vi "Repeater.vi"(7 "Name":string="Repeater", 10 "Finish On":T1, 11 "Node In":refnum<class "abs_Node.lvclass">) -> (3 "Node Out":refnum<class "abs_Node.lvclass">)   [LabVIEW 2021, in "BT.lvlib"]
uses:
  BT.lvlib
  abs_Node/abs_Node.lvclass
  Repeater/Support/Finish On - Type.ctl
  Repeater/Repeater.lvclass
  C:/Users/Tim/Documents/LabVIEW/2021/Behaviour Tree/abs_Node/abs_Node.lvclass
  C:/Users/Tim/Documents/LabVIEW/2021/Behaviour Tree/abs_Decorator/abs_Decorator.lvclass
  abs_Node/abs_Node.lvclass/abs_Node.ctl
  abs_Decorator/abs_Decorator.lvclass/abs_Decorator.ctl
  Repeater/Repeater.lvclass/Repeater.ctl
  abs_Node/Properties/Write Name.vi
  abs_Decorator/Properties/Write Node.vi
  Repeater/Properties/Write Finish On.vi
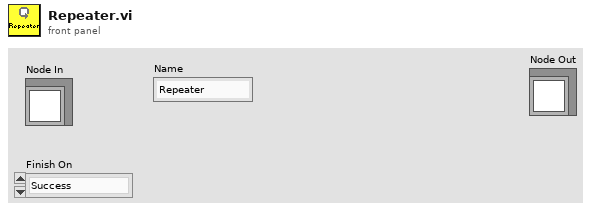
[diagram p1: front panel]
types:
  T1 = typedef "BT.lvlib/Repeater.lvclass/Finish On - Type.ctl" = enum16{"Success", "Failure", "Never"}
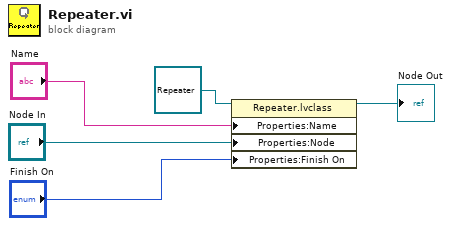
[diagram p0: block diagram]
diagram:
  n1 = property class="Repeater.lvclass"(reference=refnum<class "Repeater.lvclass"> refnum ("BT.lvlib:Repeater.lvclass"), "Properties:Name"="Name", "Properties:Node"="Node In", "Properties:Finish On"="Finish On") -> (reference out=→"Node Out":refnum<class "Repeater.lvclass">)  [unwired: 1 in, 1 out]
